vi "Begin.vi"(8 "error in":errorcluster) -> (0 "error out":errorcluster)   [LabVIEW 2016]
doc: "Called before other user functions, this VI is expected to open initial I/O refnums, load in file data, and do all program initialization. Notice that the <B>error out</B> terminal is simply used for data flow. Wiring it to other structures or subVIs ensures that this VI runs first."
uses:
  <vilib>/Rock Robotics/WPI/SafetyOutput/WPI_SafetyOutputConfigMenu.ctl
  <vilib>/Rock Robotics/WPI/DriverStation/WPI_DriverStationRobotMode2.ctl
  <vilib>/Rock Robotics/WPI/Joystick/WPI_JoystickDeviceEnum.ctl
  <vilib>/Rock Robotics/WPI/Solenoid/WPI_SolenoidChannel.ctl
  <vilib>/Rock Robotics/SystemInterfaces/DIO/FPGA_DIOChannel.ctl
  <vilib>/Rock Robotics/WPI/ThirdParty/CanMotor/TalonSRX/WPI_CANTalonSRX_BrakeOverride.ctl
  <vilib>/Rock Robotics/SystemInterfaces/spilib/spi_bus.ctl
  <vilib>/Rock Robotics/WPI/Encoder/WPI_EncoderType.ctl
  <vilib>/Rock Robotics/SystemInterfaces/DIO/FPGA_DIORelayChannel.ctl
  <vilib>/Rock Robotics/WPI/Relay/WPI_RelayDirection.ctl
  <vilib>/Rock Robotics/WPI/Solenoid/WPI_SolenoidValue.ctl
  Robot Global Data.vi
  <vilib>/Rock Robotics/Network Tables/NT Write String Array.vi
  <vilib>/Rock Robotics/WPI/Solenoid/WPI_SolenoidOpenDouble.vi
  <vilib>/Rock Robotics/WPI/Counter/WPI_CounterDigitalInputToDigitalSource.vi
  <vilib>/Rock Robotics/WPI/Gyro/WPI_GyroXRS450_SPI_Open.vi
  <vilib>/Rock Robotics/WPI/Solenoid/WPI_SolenoidSetEnum.vi
  <vilib>/Rock Robotics/WPI/RobotDrive/WPI_RobotDriveOpen4MotorWithExistingMotors.vi
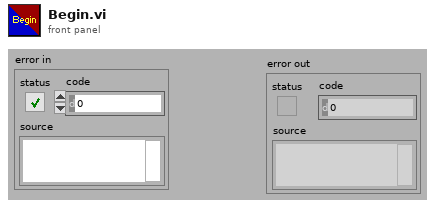
[diagram p1: front panel]
types:
  T1 = typedef "FPGA_DIOChannel.ctl" = enum8{"DIO 0", "DIO 1", "DIO 2", "DIO 3", "DIO 4", "DIO 5", "DIO 6", "DIO 7", "DIO 8", "DIO 9", "DIO MXP 0", "DIO MXP 1", "DIO MXP 2", "DIO MXP 3", "DIO MXP 4", "DIO MXP 5", "DIO MXP 6", "DIO MXP 7", "DIO MXP 8", "DIO MXP 9", "DIO MXP 10", "DIO MXP 11", "DIO MXP 12", "DIO MXP 13", "DIO MXP 14", "DIO MXP 15", "SPI Port CS1", "SPI Port CS2", "SPI Port CS3", "SPI Port MISO", "SPI Port MOSI", "Invalid"}
  T2 = typedef "WPI_SolenoidValue.ctl" = enum16{"Off", "On", "Forward", "Reverse"}
  T3 = typedef "WPI_CANTalonSRX_BrakeOverride.ctl" = enum8{"No Override", "Override to Coast", "Override to Brake"}
  T4 = typedef "WPI_RelayDirection.ctl" = enum16{"Both directions", "Forward only", "Reverse only"}
  T5 = typedef "FPGA_DIORelayChannel.ctl" = enum8{"Relay 0", "Relay 1", "Relay 2", "Relay 3", "Invalid"}
  T6 = typedef "WPI_EncoderType.ctl" = enum16{"1x", "2x", "4x"}
  T7 = typedef "WPI_SolenoidChannel.ctl" = enum8{"Solenoid 0", "Solenoid 1", "Solenoid 2", "Solenoid 3", "Solenoid 4", "Solenoid 5", "Solenoid 6", "Solenoid 7", "Invalid"}
  T8 = typedef "spi_bus.ctl" = enum16{"SPI On-Board, CS0", "SPI On-Board, CS1", "SPI On-Board, CS2", "SPI On-Board, CS3", "SPI MXP", "Invalid"}
  T9 = typedef "WPI_JoystickDeviceEnum.ctl" = enum16{"USB 0", "USB 1", "USB 2", "USB 3", "USB 4", "USB 5"}
  T10 = typedef "WPI_DriverStationRobotMode2.ctl" = enum16{"Autonomous Disabled", "Autonomous Enabled", "Teleop Disabled", "Teleop Enabled", "Disconnected", "Finish", "Test Disabled", "Test Enabled", "Emergency Stopped"}
  T11 = typedef "WPI_SafetyOutputConfigMenu.ctl" = enum16{"Enable", "Disable"}
  T12 = typedef "WPI_DigitalInputDevRef.ctl" = cluster{"DevStatus":errorcluster, "DIO Channel":T1}
  T13 = typedef "WPI_JoystickDevRef.ctl" = cluster{"Device":T9}
  T14 = typedef "WPI_MotorControlDeviceRef.ctl" = cluster{"DeviceStatus":errorcluster, "Type":T15, "PWM":cluster{"PWM Channel":T16, "DeadBand":T17}, "CAN":cluster{"Device Number":u8, "SetOutput VI Ref":variant, "GetOutput VI Ref":variant, "Enable VI Ref":variant, "Disable VI Ref":variant, "Data":variant}, "Invert":bool}
  T15 = typedef "WPI_MotorControlType.ctl" = enum16{"PWM", "CAN"}
  T16 = typedef "FPGA_DIOPWMChannel.ctl" = enum8{"PWM 0", "PWM 1", "PWM 2", "PWM 3", "PWM 4", "PWM 5", "PWM 6", "PWM 7", "PWM 8", "PWM 9", "PWM MXP 0", "PWM MXP 1", "PWM MXP 2", "PWM MXP 3", "PWM MXP 4", "PWM MXP 5", "PWM MXP 6", "PWM MXP 7", "PWM MXP 8", "PWM MXP 9", "Invalid"}
  T17 = typedef "WPI_PWMDeadband.ctl" = cluster{"Name":string, "maxPositivePwm":i32, "minPositivePwm":i32, "centerPwm":i32, "maxNegativePwm":i32, "minNegativePwm":i32, "angularRange":u16}
  T18 = typedef "FPGA_CounterEncoderSourceConvertionLVSourceType.ctl" = cluster{"DevStatus":errorcluster, "AnalogTriggerMode?":bool, "DigitalMode":cluster{"DIO Channel":T19}, "AnalogTriggerMode":cluster{"AnalogTriggerIndex":T20, "OutputType":T21}}
  T19 = typedef "FPGA_DIODigitalSourceChannel.ctl" = enum8{"DIO 0", "DIO 1", "DIO 2", "DIO 3", "DIO 4", "DIO 5", "DIO 6", "DIO 7", "DIO 8", "DIO 9", "DIO MXP 0", "DIO MXP 1", "DIO MXP 2", "DIO MXP 3", "DIO MXP 4", "DIO MXP 5", "DIO MXP 6", "DIO MXP 7", "DIO MXP 8", "DIO MXP 9", "DIO MXP 10", "DIO MXP 11", "DIO MXP 12", "DIO MXP 13", "DIO MXP 14", "DIO MXP 15", "Disabled"}
  T20 = typedef "FPGA_AnalogTriggerIndex.ctl" = enum8{"Trig 0", "Trig 1", "Trig 2", "Trig 3", "Trig 4", "Trig 5", "Trig 6", "Trig 7", "Invalid"}
  T21 = typedef "FPGA_AnalogTriggerOutType.ctl" = enum16{"InWindow", "TriggerState", "Rising", "Falling"}
  T22 = typedef "WPI_RelayDevRef.ctl" = cluster{"DevStatus":errorcluster, "Relay Channel":T5, "Relay Direction":T4}
  T23 = typedef "WPI_SolenoidDevRef.ctl" = cluster{"DevStatus":errorcluster, "Pneumatics Control Module":u8, "Forward Solenoid Channel":T7, "Reverse Solenoid Channel":T7}
  T24 = typedef "WPI_EncoderDevRef.ctl" = cluster{"DevStatus":errorcluster, "EncoderIndex":T25, "CounterIndex":T26, "DistancePerCount":dbl, "Decoding Type":T6}
  T25 = typedef "FPGA_EncoderIdx.ctl" = enum8{"Enc 0", "Enc 1", "Enc 2", "Enc 3", "Enc 4", "Enc 5", "Enc 6", "Enc 7", "Invalid"}
  T26 = typedef "FPGA_CounterCtrSystemIndex.ctl" = enum8{"Ctr 0", "Ctr 1", "Ctr 2", "Ctr 3", "Ctr 4", "Ctr 5", "Ctr 6", "Ctr 7", "Invalid"}
  T27 = typedef "WPI_GyroDevRef.ctl" = cluster{"DevStatus":errorcluster, "Analog Channel":T28, "Offset":dbl, "Gain (VoltsPerDegree/Second)":dbl, "Gyro Type":enum16{"Analog", "XRS450"}, "Handle":i32, "SPI Bus":T8, "Device Found":bool, "Sample Rate":dbl, "Calibrate On Open":bool}
  T28 = typedef "FPGA_AIChannel.ctl" = enum8{"AI 0", "AI 1", "AI 2", "AI 3", "AI MXP 0", "AI MXP 1", "AI MXP 2", "AI MXP 3", "Invalid"}
  T29 = typedef "WPI_RobotDriveDevRef.ctl" = cluster{"DevStatus":errorcluster, "Motors[]":T14[], "Square Inputs":bool, "Max Output":dbl}
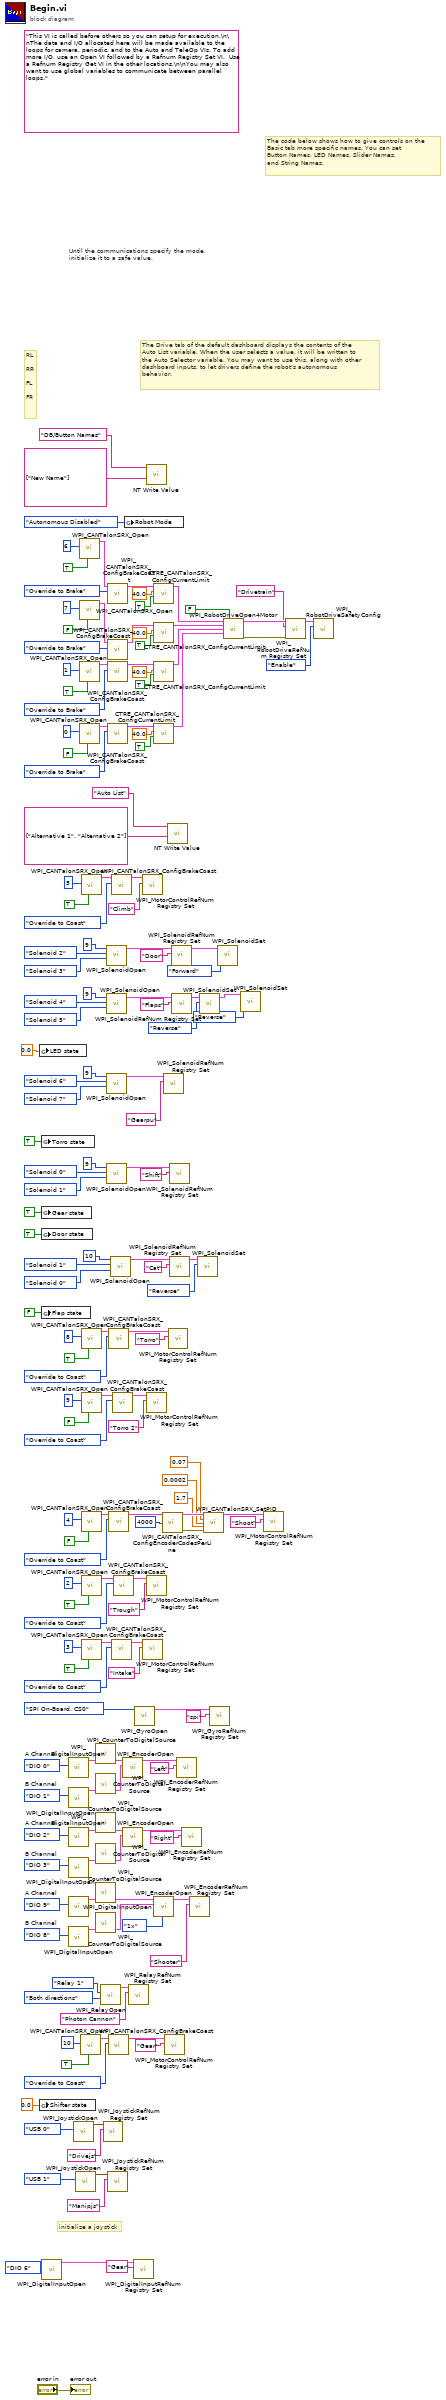
[diagram p0: block diagram]
diagram:
  w67 = FPGA_DIOChannel."DIO 8"  # B Channel
  w66 = FPGA_DIOChannel."DIO 9"  # A Channel
  w120 = FPGA_DIOChannel."DIO 3"  # B Channel
  w119 = FPGA_DIOChannel."DIO 2"  # A Channel
  w126 = FPGA_DIOChannel."DIO 1"  # B Channel
  w125 = FPGA_DIOChannel."DIO 0"  # A Channel
  (unwired) "This VI is called before others so you can setup for execution.\n\nThe data and I/O allocated here will be made available to the loops for camera, periodic, and to the Auto and TeleOp VIs. To add more I/O, use an Open VI followed by a Refnum Registry Set VI.  Use a Refnum Registry Get VI in the other locations.\n\nYou may also want to use global variables to communicate between parallel loops."
  # "RL\n\nRR\n\nFL\n\nFR"
  # "The Drive tab of the default dashboard displays the contents of the\nAuto List variable. When the user selects a value, it will be written to\nthe Auto Selector variable. You may want to use this, along with other\ndashboard inputs, to let drivers define the robot's autonomous\nbehavior."
  # "The code below shows how to give controls on the\nBasic tab more specific names. You can set\nButton Names, LED Names, Slider Names,\nand String Names."
  # "initialize a joystick"
  # "Until the communications specify the mode,\ninitialize it to a safe value."
  n1 = global write "Robot Global Data.vi" "LED state"(0.0 ("LED state")) -> ()
  n2 = global write "Robot Global Data.vi" "Shifter state"(0.0 ("Shifter state")) -> ()
  n3 = global write "Robot Global Data.vi" "Torro state"(TRUE ("Torro state")) -> ()
  n4 = global write "Robot Global Data.vi" "Gear state"(TRUE ("Torro state")) -> ()
  n5 = global write "Robot Global Data.vi" "Door state"(TRUE ("Door state")) -> ()
  n6 = global write "Robot Global Data.vi" "Flap state"(FALSE ("Flap state")) -> ()
  n7 = call <vilib>:"WPI_DigitalInputOpen.vi"("DIO Channel"=FPGA_DIOChannel."DIO 6") -> ("DigitalInputDevRef"=w2:T12)  [unwired: 9 in, 1 out]
  n8 = call <vilib>:"WPI_DigitalInputOpen.vi"("DIO Channel"=w125) -> ("DigitalInputDevRef"=w122:T12)  [unwired: 1 in, 9 out]
  n9 = call <vilib>:"WPI_DigitalInputOpen.vi"("DIO Channel"=w126) -> ("DigitalInputDevRef"=w123:T12)  [unwired: 1 in, 9 out]
  n10 = call <vilib>:"WPI_DigitalInputOpen.vi"("DIO Channel"=w119) -> ("DigitalInputDevRef"=w116:T12)  [unwired: 1 in, 9 out]
  n11 = call <vilib>:"WPI_DigitalInputOpen.vi"("DIO Channel"=w120) -> ("DigitalInputDevRef"=w117:T12)  [unwired: 1 in, 9 out]
  n12 = call <vilib>:"WPI_DigitalInputOpen.vi"("DIO Channel"=w66) -> ("DigitalInputDevRef"=w63:T12)  [unwired: 1 in, 9 out]
  n13 = call <vilib>:"WPI_DigitalInputOpen.vi"("DIO Channel"=w67) -> ("DigitalInputDevRef"=w64:T12)  [unwired: 1 in, 9 out]
  n14 = call <vilib>:"WPI_JoystickOpen.vi"("JoystickDevice"=WPI_JoystickDeviceEnum."USB 0") -> ("JoystickDevRef"=w167:T13)  [unwired: 10 in]
  n15 = call <vilib>:"WPI_JoystickOpen.vi"("JoystickDevice"=WPI_JoystickDeviceEnum."USB 1") -> ("JoystickDevRef"=w98:T13)  [unwired: 10 in]
  n16 = call <vilib>:"WPI_CANTalonSRX_Open.vi"("Invert"=TRUE, "Device Number"=u8 6) -> ("CAN Talon SRX Ref"=w85:T14)  [unwired: 8 in, 1 out]
  n17 = call <vilib>:"WPI_CANTalonSRX_Open.vi"("Invert"=FALSE, "Device Number"=u8 7) -> ("CAN Talon SRX Ref"=w81:T14)  [unwired: 8 in, 1 out]
  n18 = call <vilib>:"WPI_CANTalonSRX_Open.vi"("Invert"=TRUE, "Device Number"=u8 1) -> ("CAN Talon SRX Ref"=w80:T14)  [unwired: 8 in, 1 out]
  n19 = call <vilib>:"WPI_CANTalonSRX_Open.vi"("Invert"=FALSE, "Device Number"=u8 0) -> ("CAN Talon SRX Ref"=w79:T14)  [unwired: 8 in, 1 out]
  n20 = call <vilib>:"WPI_CANTalonSRX_Open.vi"("Invert"=TRUE, "Device Number"=u8 10) -> ("CAN Talon SRX Ref"=w11:T14)  [unwired: 8 in, 1 out]
  n21 = call <vilib>:"WPI_CANTalonSRX_Open.vi"("Invert"=TRUE, "Device Number"=u8 5) -> ("CAN Talon SRX Ref"=w149:T14)  [unwired: 8 in, 1 out]
  n22 = call <vilib>:"WPI_CANTalonSRX_Open.vi"("Invert"=TRUE, "Device Number"=u8 8) -> ("CAN Talon SRX Ref"=w55:T14)  [unwired: 8 in, 1 out]
  n23 = call <vilib>:"WPI_CANTalonSRX_Open.vi"("Invert"=FALSE, "Device Number"=u8 9) -> ("CAN Talon SRX Ref"=w38:T14)  [unwired: 8 in, 1 out]
  n24 = call <vilib>:"WPI_CANTalonSRX_Open.vi"("Invert"=FALSE, "Device Number"=u8 4) -> ("CAN Talon SRX Ref"=w134:T14)  [unwired: 8 in, 1 out]
  n25 = call <vilib>:"WPI_CANTalonSRX_Open.vi"("Invert"=TRUE, "Device Number"=u8 2) -> ("CAN Talon SRX Ref"=w129:T14)  [unwired: 8 in, 1 out]
  n26 = call <vilib>:"WPI_CANTalonSRX_Open.vi"("Invert"=TRUE, "Device Number"=u8 3) -> ("CAN Talon SRX Ref"=w107:T14)  [unwired: 8 in, 1 out]
  n27 = call-poly <vilib>:"WPI_CounterToDigitalSource.vi"("DigitalInputDevRef"=w122) -> ("Digital Source"=w121:T18)  [unwired: 6 out]
  n28 = call-poly <vilib>:"WPI_CounterToDigitalSource.vi"("DigitalInputDevRef"=w123) -> ("Digital Source"=w124:T18)  [unwired: 6 out]
  n29 = call-poly <vilib>:"WPI_CounterToDigitalSource.vi"("DigitalInputDevRef"=w116) -> ("Digital Source"=w115:T18)  [unwired: 6 out]
  n30 = call-poly <vilib>:"WPI_CounterToDigitalSource.vi"("DigitalInputDevRef"=w117) -> ("Digital Source"=w118:T18)  [unwired: 6 out]
  n31 = call-poly <vilib>:"WPI_CounterToDigitalSource.vi"("DigitalInputDevRef"=w63) -> ("Digital Source"=w62:T18)  [unwired: 6 out]
  n32 = call-poly <vilib>:"WPI_CounterToDigitalSource.vi"("DigitalInputDevRef"=w64) -> ("Digital Source"=w65:T18)  [unwired: 6 out]
  n33 = call <vilib>:"WPI_RelayOpen.vi"("Relay Direction"=WPI_RelayDirection."Both directions", "Relay Channel"=FPGA_DIORelayChannel."Relay 1") -> ("RelayDevRef"=w41:T22)  [unwired: 8 in, 1 out]
  n34 = call <vilib>:"WPI_JoystickRefNum Registry Set.vi"("refnum name"="Drivejs", "JoystickDevRef"=w167) -> ()  [unwired: 8 in, 2 out]
  n35 = call-poly <vilib>:"WPI_SolenoidOpen.vi"("Reverse Solenoid Channel"=WPI_SolenoidChannel."Solenoid 3", "Forward Solenoid Channel"=WPI_SolenoidChannel."Solenoid 2" ("Solenoid Channel"), "Pneumatics Control Module (0)"=u8 9) -> ("SolenoidDevRef"=w143:T23)  [unwired: 7 in, 1 out]
  n36 = call-poly <vilib>:"WPI_SolenoidOpen.vi"("Reverse Solenoid Channel"=WPI_SolenoidChannel."Solenoid 5", "Forward Solenoid Channel"=WPI_SolenoidChannel."Solenoid 4", "Pneumatics Control Module (0)"=u8 9) -> ("SolenoidDevRef"=w138:T23)  [unwired: 7 in, 1 out]
  n37 = call-poly <vilib>:"WPI_SolenoidOpen.vi"("Reverse Solenoid Channel"=WPI_SolenoidChannel."Solenoid 7", "Forward Solenoid Channel"=WPI_SolenoidChannel."Solenoid 6", "Pneumatics Control Module (0)"=u8 9) -> ("SolenoidDevRef"=w101:T23)  [unwired: 7 in, 1 out]
  n38 = call-poly <vilib>:"WPI_SolenoidOpen.vi"("Reverse Solenoid Channel"=WPI_SolenoidChannel."Solenoid 1", "Forward Solenoid Channel"=WPI_SolenoidChannel."Solenoid 0", "Pneumatics Control Module (0)"=u8 9) -> ("SolenoidDevRef"=w90:T23)  [unwired: 7 in, 1 out]
  n39 = call <vilib>:"WPI_CANTalonSRX_ConfigBrakeCoast.vi"("Brake / Coast Mode"=WPI_CANTalonSRX_BrakeOverride."Override to Brake", "CAN Talon SRX Ref"=w85) -> ("CAN Talon SRX Ref"=w16:T14)  [unwired: 8 in, 1 out]
  n40 = call <vilib>:"WPI_CANTalonSRX_ConfigBrakeCoast.vi"("Brake / Coast Mode"=WPI_CANTalonSRX_BrakeOverride."Override to Brake", "CAN Talon SRX Ref"=w81) -> ("CAN Talon SRX Ref"=w20:T14)  [unwired: 8 in, 1 out]
  n41 = call <vilib>:"WPI_CANTalonSRX_ConfigBrakeCoast.vi"("Brake / Coast Mode"=WPI_CANTalonSRX_BrakeOverride."Override to Brake", "CAN Talon SRX Ref"=w80) -> ("CAN Talon SRX Ref"=w24:T14)  [unwired: 8 in, 1 out]
  n42 = call <vilib>:"WPI_CANTalonSRX_ConfigBrakeCoast.vi"("Brake / Coast Mode"=WPI_CANTalonSRX_BrakeOverride."Override to Brake", "CAN Talon SRX Ref"=w79) -> ("CAN Talon SRX Ref"=w30:T14)  [unwired: 8 in, 1 out]
  n43 = call <vilib>:"WPI_JoystickRefNum Registry Set.vi"("refnum name"="Manipjs", "JoystickDevRef"=w98) -> ()  [unwired: 8 in, 2 out]
  n44 = call <vilib>:"WPI_CANTalonSRX_ConfigBrakeCoast.vi"("Brake / Coast Mode"=WPI_CANTalonSRX_BrakeOverride."Override to Coast", "CAN Talon SRX Ref"=w11) -> ("CAN Talon SRX Ref"=w10:T14)  [unwired: 8 in, 1 out]
  n45 = call <vilib>:"WPI_CANTalonSRX_ConfigBrakeCoast.vi"("Brake / Coast Mode"=WPI_CANTalonSRX_BrakeOverride."Override to Coast", "CAN Talon SRX Ref"=w55) -> ("CAN Talon SRX Ref"=w51:T14)  [unwired: 8 in, 1 out]
  n46 = call <vilib>:"WPI_CANTalonSRX_ConfigBrakeCoast.vi"("Brake / Coast Mode"=WPI_CANTalonSRX_BrakeOverride."Override to Coast", "CAN Talon SRX Ref"=w134) -> ("CAN Talon SRX Ref"=w58:T14)  [unwired: 8 in, 1 out]
  n47 = call-poly <vilib>:"WPI_SolenoidOpen.vi"("Reverse Solenoid Channel"=WPI_SolenoidChannel."Solenoid 0", "Forward Solenoid Channel"=WPI_SolenoidChannel."Solenoid 1", "Pneumatics Control Module (0)"=u8 10) -> ("SolenoidDevRef"=w72:T23)  [unwired: 7 in, 1 out]
  n48 = call <vilib>:"WPI_CANTalonSRX_ConfigBrakeCoast.vi"("Brake / Coast Mode"=WPI_CANTalonSRX_BrakeOverride."Override to Coast", "CAN Talon SRX Ref"=w149) -> ("CAN Talon SRX Ref"=w148:T14)  [unwired: 8 in, 1 out]
  n49 = call <vilib>:"WPI_CANTalonSRX_ConfigBrakeCoast.vi"("Brake / Coast Mode"=WPI_CANTalonSRX_BrakeOverride."Override to Coast", "CAN Talon SRX Ref"=w107) -> ("CAN Talon SRX Ref"=w106:T14)  [unwired: 8 in, 1 out]
  n50 = call <vilib>:"WPI_CANTalonSRX_ConfigBrakeCoast.vi"("Brake / Coast Mode"=WPI_CANTalonSRX_BrakeOverride."Override to Coast", "CAN Talon SRX Ref"=w38) -> ("CAN Talon SRX Ref"=w34:T14)  [unwired: 8 in, 1 out]
  n51 = call <vilib>:"WPI_CANTalonSRX_ConfigBrakeCoast.vi"("Brake / Coast Mode"=WPI_CANTalonSRX_BrakeOverride."Override to Coast", "CAN Talon SRX Ref"=w129) -> ("CAN Talon SRX Ref"=w128:T14)  [unwired: 8 in, 1 out]
  n52 = call <vilib>:"WPI_EncoderOpen.vi"("BSource"=w124, "ASource"=w121) -> ("EncoderDevRef"=w114:T24)  [unwired: 6 in, 3 out]
  n53 = call <vilib>:"WPI_EncoderOpen.vi"("BSource"=w118, "ASource"=w115) -> ("EncoderDevRef"=w112:T24)  [unwired: 6 in, 3 out]
  n54 = global write "Robot Global Data.vi" "Robot Mode"(WPI_DriverStationRobotMode2."Autonomous Disabled" ("Robot Mode")) -> ()
  n55 = call <vilib>:"WPI_RelayRefNum Registry Set.vi"("refnum name"="Photon Cannon", "RelayDevRef"=w41) -> ()  [unwired: 8 in, 2 out]
  n56 = call <vilib>:"WPI_DigitalInputRefNum Registry Set.vi"("refnum name"="Gear", "DigitalInputDevRef"=w2) -> ()  [unwired: 8 in, 2 out]
  n57 = call-poly <vilib>:"WPI_GyroOpen.vi"("SPI Bus"=spi_bus."SPI On-Board, CS0") -> ("GyroDevRef"=w95:T27)  [unwired: 9 in, 1 out]
  n58 = call <vilib>:"WPI_MotorControlRefNum Registry Set.vi"("refnum name"="Climb", "MotorControlDevRef"=w148) -> ()  [unwired: 8 in, 2 out]
  n59 = call <vilib>:"WPI_MotorControlRefNum Registry Set.vi"("refnum name"="Intake", "MotorControlDevRef"=w106) -> ()  [unwired: 8 in, 2 out]
  n60 = call-poly <vilib>:"NT Write Value.vi"("String Array"=string[] ["New Name"], "Name"="DB/Button Names") -> ()  [unwired: 9 in, 1 out]
  n61 = call <vilib>:"WPI_MotorControlRefNum Registry Set.vi"("refnum name"="Torro 2", "MotorControlDevRef"=w34) -> ()  [unwired: 8 in, 2 out]
  n62 = call <vilib>:"WPI_MotorControlRefNum Registry Set.vi"("refnum name"="Trough", "MotorControlDevRef"=w128) -> ()  [unwired: 8 in, 2 out]
  n63 = call <vilib>:"CTRE_CANTalonSRX_ConfigCurrentLimit.vi"("Enable Current Limit?"=TRUE, "Current Limit (Amps)"=40.0, "CAN Talon SRX Ref"=w16) -> ("CAN Talon SRX Ref 2"=w15:T14)  [unwired: 7 in, 1 out]
  n64 = call <vilib>:"CTRE_CANTalonSRX_ConfigCurrentLimit.vi"("Enable Current Limit?"=TRUE, "Current Limit (Amps)"=40.0, "CAN Talon SRX Ref"=w20) -> ("CAN Talon SRX Ref 2"=w19:T14)  [unwired: 7 in, 1 out]
  n65 = call <vilib>:"CTRE_CANTalonSRX_ConfigCurrentLimit.vi"("Enable Current Limit?"=TRUE, "Current Limit (Amps)"=40.0, "CAN Talon SRX Ref"=w24) -> ("CAN Talon SRX Ref 2"=w23:T14)  [unwired: 7 in, 1 out]
  n66 = call <vilib>:"CTRE_CANTalonSRX_ConfigCurrentLimit.vi"("Enable Current Limit?"=TRUE, "Current Limit (Amps)"=40.0, "CAN Talon SRX Ref"=w30) -> ("CAN Talon SRX Ref 2"=w29:T14)  [unwired: 7 in, 1 out]
  n67 = call <vilib>:"WPI_EncoderOpen.vi"("Decoding Type"=WPI_EncoderType."1x", "BSource"=w65, "ASource"=w62) -> ("EncoderDevRef"=w59:T24)  [unwired: 5 in, 3 out]
  n68 = call <vilib>:"WPI_CANTalonSRX_ConfigEncoderCodesPerLine.vi"("CAN Talon SRX Ref"=w58, "Number Encoder Lines\n(Counts Per Rotation)"=u32 4000 ("Number Encoder Lines\n(Counts Per Rotation)")) -> ("CAN Talon SRX Ref"=w50:T14, "error out"=w49:errorcluster)  [unwired: 12 in]
  n69 = call <vilib>:"WPI_SolenoidRefNum Registry Set.vi"("refnum name"="Gearpu", "SolenoidDevRef"=w101) -> ()  [unwired: 8 in, 2 out]
  n70 = call <vilib>:"WPI_MotorControlRefNum Registry Set.vi"("refnum name"="Gear", "MotorControlDevRef"=w10) -> ()  [unwired: 8 in, 2 out]
  n71 = call-poly <vilib>:"NT Write Value.vi"("String Array"=string[] ["Alternative 1", "Alternative 2"], "Name"="Auto List") -> ()  [unwired: 9 in, 1 out]
  n72 = call <vilib>:"WPI_MotorControlRefNum Registry Set.vi"("refnum name"="Torro", "MotorControlDevRef"=w51) -> ()  [unwired: 8 in, 2 out]
  n73 = call <vilib>:"WPI_SolenoidRefNum Registry Set.vi"("refnum name"="Shift", "SolenoidDevRef"=w90) -> ()  [unwired: 8 in, 2 out]
  n74 = call <vilib>:"WPI_SolenoidRefNum Registry Set.vi"("refnum name"="Cat", "SolenoidDevRef"=w72) -> ("SolenoidDevRef"=w70:T23)  [unwired: 8 in, 1 out]
  n75 = call <vilib>:"WPI_SolenoidRefNum Registry Set.vi"("refnum name"="Door", "SolenoidDevRef"=w143) -> ("SolenoidDevRef"=w5:T23)  [unwired: 8 in, 1 out]
  n76 = call <vilib>:"WPI_SolenoidRefNum Registry Set.vi"("refnum name"="Flaps", "SolenoidDevRef"=w138) -> ("SolenoidDevRef"=w77:T23)  [unwired: 8 in, 1 out]
  n77 = call <vilib>:"WPI_EncoderRefNum Registry Set.vi"("refnum name"="Left", "EncoderDevRef"=w114) -> ()  [unwired: 8 in, 2 out]
  n78 = call <vilib>:"WPI_EncoderRefNum Registry Set.vi"("refnum name"="Right", "EncoderDevRef"=w112) -> ()  [unwired: 8 in, 2 out]
  n79 = call <vilib>:"WPI_EncoderRefNum Registry Set.vi"("refnum name"="Shooter", "EncoderDevRef"=w59) -> ()  [unwired: 8 in, 2 out]
  n80 = call-poly <vilib>:"WPI_SolenoidSet.vi"("Value"=WPI_SolenoidValue."Reverse", "SolenoidDevRef"=w70) -> ()  [unwired: 8 in, 2 out]
  n81 = call-poly <vilib>:"WPI_SolenoidSet.vi"("Value"=WPI_SolenoidValue."Reverse", "SolenoidDevRef"=w77) -> ("SolenoidDevRef"=w7:T23)  [unwired: 8 in, 1 out]
  n82 = call <vilib>:"WPI_CANTalonSRX_SetPID.vi"("CAN Talon SRX Ref"=w50, "P"=0.07, "I"=0.0002, "D"=1.7, "error in (no error)"=w49) -> ("CAN Talon SRX Ref"=w45:T14)  [unwired: 9 in, 1 out]
  n83 = call <vilib>:"WPI_GyroRefNum Registry Set.vi"("refnum name"="spi", "GyroDevRef"=w95) -> ()  [unwired: 8 in, 2 out]
  n84 = call-poly <vilib>:"WPI_SolenoidSet.vi"("Value"=WPI_SolenoidValue."Forward", "SolenoidDevRef"=w5) -> ()  [unwired: 8 in, 2 out]
  n85 = call-poly <vilib>:"WPI_RobotDriveOpen4Motor.vi"("Rear Left Motor Dev Ref"=w15, "Square Inputs"=FALSE, "Rear Right Motor Dev Ref"=w19, "Front Left Motor Dev Ref"=w23, "Front Right Motor Dev Ref"=w29) -> ("RobotDriveDevRef"=w173:T29, "error out"=w172:errorcluster)  [unwired: 9 in]
  n86 = call-poly <vilib>:"WPI_SolenoidSet.vi"("Value"=WPI_SolenoidValue."Reverse", "SolenoidDevRef"=w7) -> ()  [unwired: 8 in, 2 out]
  n87 = call <vilib>:"WPI_MotorControlRefNum Registry Set.vi"("refnum name"="Shoot", "MotorControlDevRef"=w45) -> ()  [unwired: 8 in, 2 out]
  n88 = call <vilib>:"WPI_RobotDriveRefNum Registry Set.vi"("error in (no error)"=w172, "refnum name"="Drivetrain", "RobotDriveDevRef"=w173) -> ("RobotDriveDevRef"=w171:T29)  [unwired: 1 in, 7 out]
  n89 = call <vilib>:"WPI_RobotDriveSafetyConfig.vi"("mode"=WPI_SafetyOutputConfigMenu."Enable", "RobotDriveDevRef"=w171) -> ()  [unwired: 8 in, 2 out]
  "error out" <- "error in"
